vi "Save data to file.vi"(0 "current time":timestamp, 1 "Save path":path, 2 "Save":bool, 3 "RH":dbl, 4 "H2O[ppm]":dbl, 5 "Tdf['C]":dbl) -> ()   [LabVIEW 2018]
uses:
  <vilib>/Utility/file.llb/Write To Spreadsheet File (string).vi
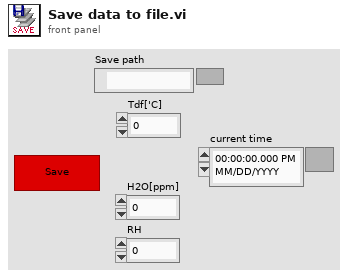
[diagram p1: front panel]
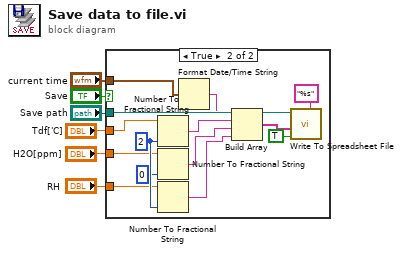
[diagram p0: block diagram]
diagram:
  n1 = case shown="True" "Save" {
    tunnel: "Save path" -> [_ w19]
    tunnel: "Tdf['C]" -> [_ w17]
    tunnel: "H2O[ppm]" -> [_ w12]
    tunnel: "RH" -> [_ w11]
    tunnel: "current time" -> [_ w9]
    frame False {
    }
    frame True {
      w16 = i16 2 ("precision (6)")
      n2 = Number To Fractional String(number=w17, precision (6)=w16) -> (F-format string=w14:string)  [unwired: 2 in]
      n3 = Number To Fractional String(number=w12, precision (6)=i16 0) -> (F-format string=w8:string)  [unwired: 2 in]
      n4 = Number To Fractional String(number=w11, precision (6)=w16) -> (F-format string=w7:string)  [unwired: 2 in]
      n5 = Format Date/Time String(seconds (now)=w9) -> (date/time string=w10:string)  [unwired: 2 in]
      n6 = Build Array(w10, w14, w8, w7) -> (w13:string[])
      n7 = call-poly <vilib>:"Write To Spreadsheet File.vi"("format (%s)"="%s", "append to file? (new file:F)"=TRUE, "1D data"=w13, "file path (dialog if empty)"=w19) -> ()  [unwired: 4 in, 1 out]
    }
  }
